vi "Pre Launch Init.vi"(8 "error in":errorcluster, 10 "FGV Name":string="PLC Ref", 11 "Sequence Context In":refnum<k7>) -> (0 "error out":errorcluster, 1 "OPC subscriptID":T2, 2 "OPC Client ref":T1, 3 "Event Registration Refnum":refnum<event-registration>, 5 "Station":string)   [LabVIEW 2021, in "OPCUA.lvlib"]
uses:
  OPCUA.lvlib
  <vilib>/OPCUA/controls/Subscription ID.ctl
  <vilib>/OPCUA/controls/OPC UA Client Refnum.ctl
  <vilib>/OPCUA/controls/Subscription Data Change.ctl
  <vilib>/OPCUA/controls/NodeId.ctl
  <vilib>/OPCUA/controls/Data Type.ctl
  <vilib>/OPCUA/controls/OPC UA StatusCode.ctl
  <vilib>/addons/TestStand/_TSUtility.llb/TestStand - Get Property Value (Number {Signed 32-bit Integer}).vi
  <vilib>/OPCUA/NI OPC UA Client.lvlib
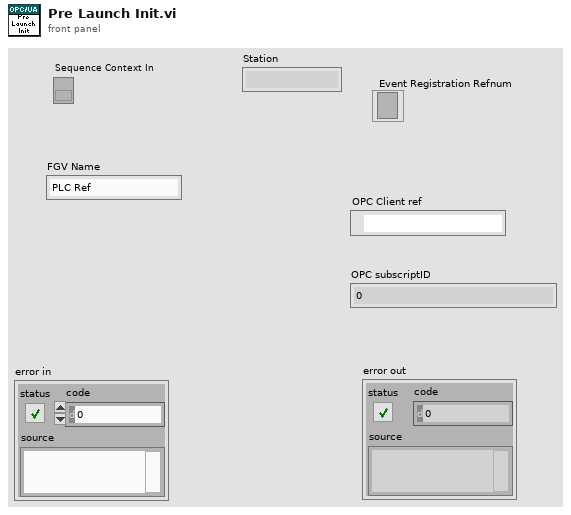
[diagram p1: front panel]
types:
  T1 = typedef "OPC UA Client Refnum.ctl" = refnum<k21>
  T2 = typedef "Subscription ID.ctl" = u32
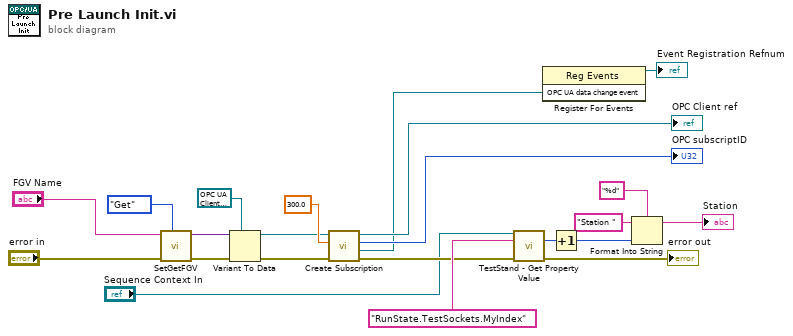
[diagram p0: block diagram]
diagram:
  n1 = call "SetGetFGV.vi"("Method (Get)"=enum16{"Get", "Set"}."Get", "error in"="error in", "FGVname"="FGV Name") -> ("error out"=w18:errorcluster, "Data out"=w21:variant)  [unwired: 7 in]
  n2 = Variant To Data(error in=w18, type=T1 refnum ("OPC UA client refnum out"), Variant=w21) -> (data=w15:T1, error out=w16:errorcluster)
  n3 = call <vilib>:"Create Subscription.vi"("error in (no error)"=w16, "publishing interval (1000 ms)"=300.0, "OPC UA client refnum in"=w15) -> ("error out"=w11:errorcluster, "OPC UA data change event"=w2:refnum<user-event>, "subscription ID out"=→"OPC subscriptID":T2, "OPC UA client refnum out"=→"OPC Client ref":T1)  [unwired: 4 in, 1 out]
  n4 = call-poly <vilib>:"TestStand - Get Property Value.vi"("Sequence Context In"="Sequence Context In", "Lookup String"="RunState.TestSockets.MyIndex", "error in (no error)"=w11) -> ("Value"=w8:i32, "error out"=→"error out":errorcluster)  [unwired: 10 in, 1 out]
  n5 = register-events(w2) -> (reference out=→"Event Registration Refnum":refnum<event-registration>)  [unwired: 2 in, 1 out]
  n6 = Increment(x=w8) -> (x+1=w4:i32)
  n7 = Format Into String(format string="%d", initial string="Station ", w4) -> (resulting string=→"Station":string)  [unwired: 1 in, 1 out]
